vi "SRLATCH.vi"(4 "Reset":bool, 8 "Set":bool) -> (0 "Output":bool)   [LabVIEW 2015]
doc: "When S is given an input of true, this VI will be set on; it will stay true as long as it is set. The VI resets when the R input turns on; it will then return false and wait for S to turn on again.\n\nIf both inputs are true, the Set is given priority and the input is set to true."
uses:
  <vilib>/functionblocks/Bistables/SR Bistable/SR Bistable.vi
  <vilib>/functionblocks/FB Core/FB Core.xnode
  <vilib>/functionblocks/NI_FunctionBlock Libraries.lvlib
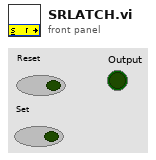
[diagram p1: front panel]
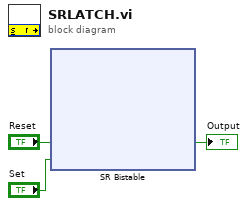
[diagram p0: block diagram]
diagram:
  n1 = xnode "SR Bistable"("reset"="Reset", "set"="Set") -> ("output"=→"Output":bool)  [unwired: 1 in, 1 out]
